vi "FIFOFileObject_old.vi"(0 "Destination:":path, 1 "buffer":u32[](array[numeric]), 2 "count":u32, 3 "error in (no error)":errorcluster, 4 "function (open:0)":enum16{"open", "write", "close"}(ring)) -> (5 "error out":errorcluster)   [LabVIEW 2009]
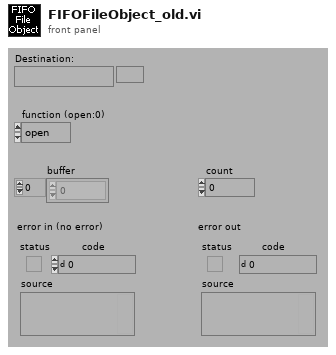
[diagram p1: front panel]
types:
  T1 = enum16{"open", "open or create", "create or replace", "create", "open (read only)"}
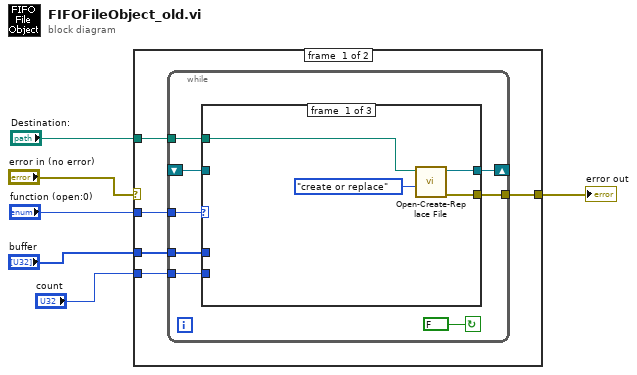
[diagram p0: block diagram]
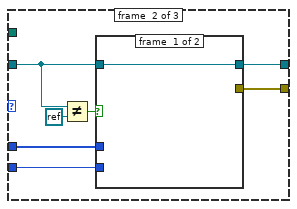
[diagram p2: hidden frame]
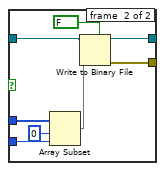
[diagram p3: hidden frame]
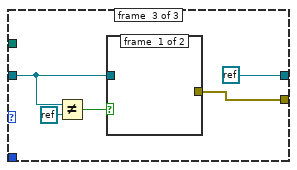
[diagram p4: hidden frame]
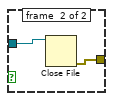
[diagram p5: hidden frame]
diagram:
  n1 = case shown="No Error" "error in (no error)" {
    selector: "error in (no error)" -> [_ w47]
    tunnel: "Destination:" -> [w11 _]
    tunnel: [w10 w47] -> w2
    tunnel: "function (open:0)" -> [w9 _]
    tunnel: "count" -> [w8 _]
    tunnel: "buffer" -> [w7 _]
    frame #0 {
      n2 = while {
        tunnel: w11 -> [w18]
        tunnel: [w17] -> w10
        shift-right: [w16] -> _
        shift-left: _ -> [w15]
        tunnel: w9 -> [w14]
        tunnel: w8 -> [w13]
        tunnel: w7 -> [w12]
        stop <- FALSE continue-if-true
        n3 = case shown="\"write\", Default" w14 {
          tunnel: w18 -> [w20 _ _]
          tunnel: [w22 w27 w43] -> w17
          tunnel: [w21 w30 refnum<k0> refnum] -> w16
          tunnel: w15 -> [_ w24 w41]
          tunnel: w13 -> [_ w29 _]
          tunnel: w12 -> [_ w28 _]
          frame #0 {
            n4 = call "Open-Create-Replace File.vi"("function (open:0)"=T1."create or replace", "file path"=w20) -> ("error out"=w22:errorcluster, "refnum"=w21:refnum<file>)  [unwired: 6 in, 2 out]
          }
          frame #1 {
            n5 = Not Equal?(x=w24, y=refnum<k0> refnum) -> (x != y?=w26:bool)
            n6 = case shown="True" w26 {
              tunnel: [w31 w37] -> w30
              tunnel: w29 -> [_ w36]
              tunnel: w28 -> [_ w35]
              tunnel: [_ w34] -> w27
              tunnel: w24 -> [w31 w33]
              frame #0 {
              }
              frame #1 {
                n7 = Array Subset(array=w35, index=0, length=w36) -> (w38:u32[])
                n8 = Write to Binary File(file (use dialog)=w33, data=w38, 5:FALSE ("prepend array or string size? (T)")) -> (refnum out=w37:refnum<file>, error out=w34:errorcluster)  [unwired: 3 in, 1 out]
              }
            }
          }
          frame #2 {
            n9 = Not Equal?(x=w41, y=refnum<k0> refnum) -> (x != y?=w40:bool)
            n10 = case shown="True" w40 {
              tunnel: [_ w46] -> w43
              tunnel: w41 -> [_ w45]
              frame #0 {
              }
              frame #1 {
                n11 = Close File(refnum=w45) -> (error out=w46:errorcluster)  [unwired: 1 in, 1 out]
              }
            }
          }
        }
      }
    }
    frame #1 {
    }
  }
  "error out" <- w2
